vi "Refresh with loaded ROI_retd.vi"(7 "ROI fit info cluster":T1 {"ROI fit info"."Frame size"."Old" items=["100X100"=100, "128X128"=128, "200X200"=200, "256X256"=256, "512X512"=512, "1024x1024"=1024, "2048x2048"=2048]; "ROI fit info"."Frame size"."New" items=["100X100"=100, "128X128"=128, "200X200"=200, "256X256"=256, "512X512"=512, "1024x1024"=1024, "2048x2048"=2048]}, 10 "Old ROI file's data":dbl[][](array[numeric]), 11 "Old ROI file path":path) -> (1 "Last ROI Enum":T3, 3 "Proceed?":bool)   [LabVIEW 2017]
uses:
  Typedefs/ROI ID Enum.ctl
  Typedefs/ROI management FG states.ctl
  Typedefs/Frame Size.ctl
  Typedefs/ROI fitting info cluster.ctl
panel:
  out "No ROI":bool
  out "Number of ROI":i32
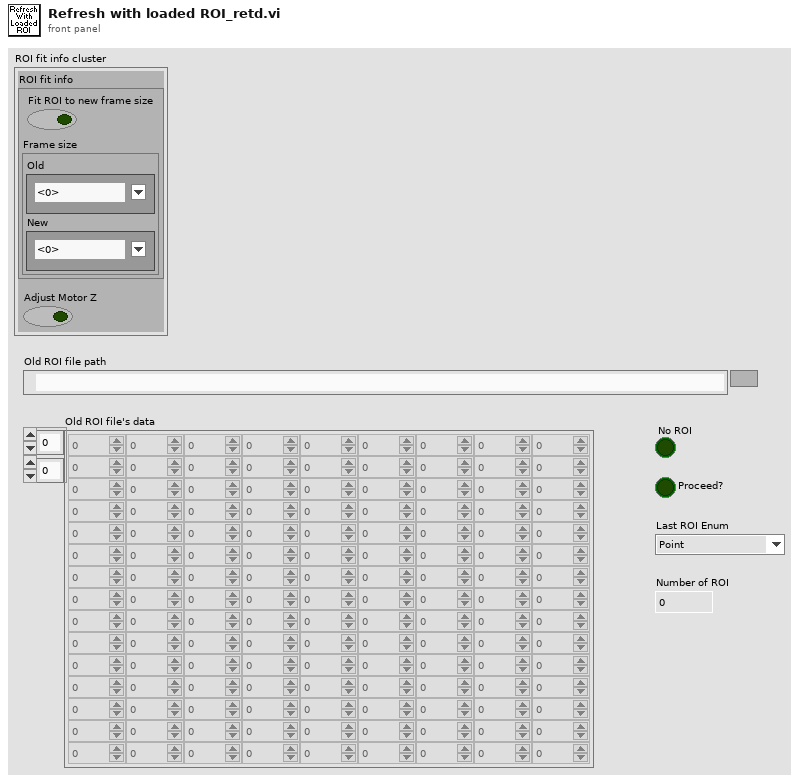
[diagram p1: front panel]
types:
  T1 = typedef "ROI fitting info cluster.ctl" = cluster{"ROI fit info":cluster{"Fit ROI to new frame size":bool, "Frame size":cluster{"Old":T2, "New":T2}}, "Adjust Motor Z":bool}
  T2 = typedef "Frame Size.ctl" = u16
  T3 = typedef "ROI ID Enum.ctl" = enum16{"Point", "MiniScan", "Comp. MiniScan", "Rectangle", "Comp. volume", "Arb. plane point"}
  T4 = typedef "ROI management FG states.ctl" = enum16{"Read", "Write", "Clear Last", "Clear All", "Update ROIs time", "Reload last ROI set", "Offset all ROI", "Offset visible ROI"}
  T5 = typedef "ROI spec.ctl" = cluster{"Coordinates":i32[], "Zoom":dbl, "ROI Enum":T3, "ZplaneIndex":i32}
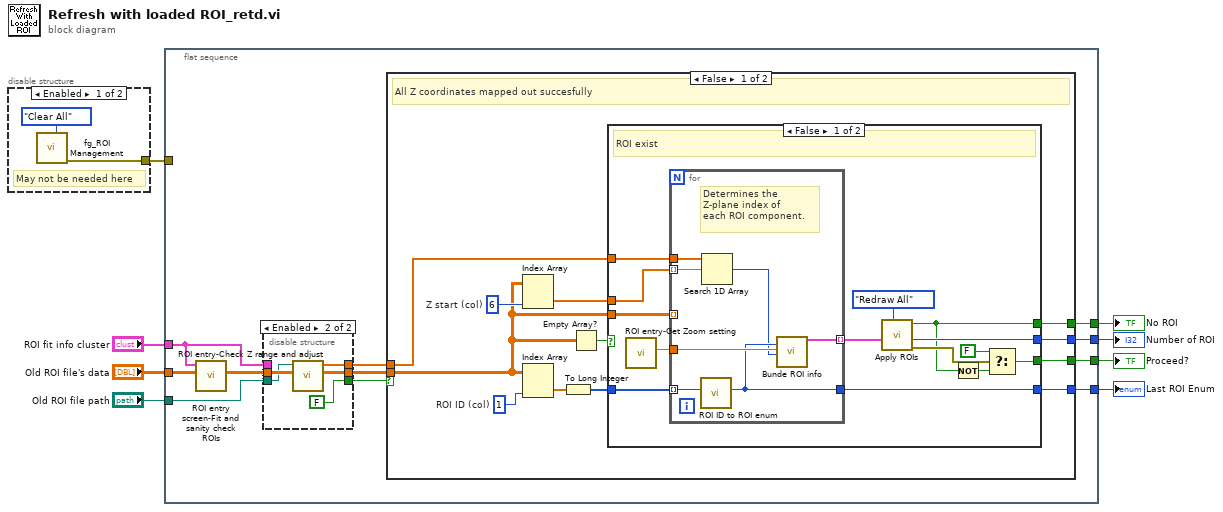
[diagram p0: block diagram]
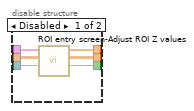
[diagram p2: hidden frame]
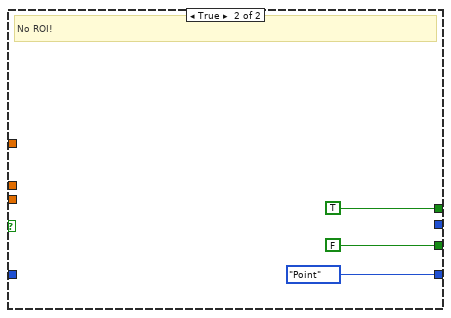
[diagram p3: hidden frame]
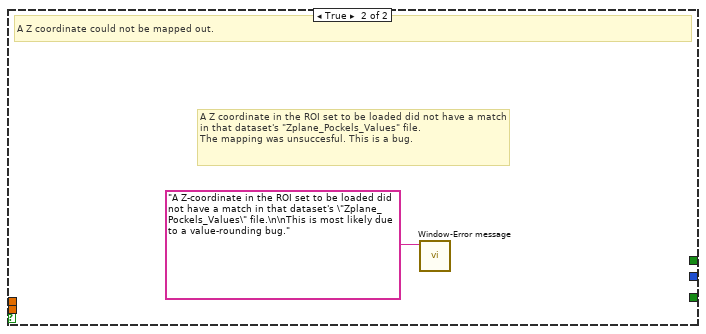
[diagram p4: hidden frame]
diagram:
  n1 = disable-structure shown="Enabled" {
    disable-tunnel: [w9 _] -> w1
    frame Enabled {
      # "May not be needed here"
      n2 = call "fg_ROI Management.vi"("Function"=ROI_management_FG_states."Clear All") -> ("error out"=w9:errorcluster)  [unwired: 6 in, 4 out]
    }
    frame Disabled {
    }
  }
  n3 = flat-sequence {
    tunnel: "Old ROI file path" -> [w13]
    tunnel: [w21] -> w7
    tunnel: [w20] -> w6
    tunnel: [w19] -> w5
    tunnel: [w18] -> w4
    tunnel: "Old ROI file's data" -> [w17]
    tunnel: "ROI fit info cluster" -> [w14]
    tunnel: w1 -> [_]
    frame #0 {
      n4 = call "ROI entry screen-Fit and sanity check ROIs.vi"("Old ROI file's data in"=w17, "ROI fit info"=w14) -> ("Fitted ROI data"=w16:dbl[][])  [unwired: 9 in]
      n5 = disable-structure shown="Enabled" {
        disable-tunnel: w16 -> [w27 w32]
        disable-tunnel: [w26 w29] -> w15
        disable-tunnel: w14 -> [w25 _]
        disable-tunnel: w13 -> [w24 w31]
        disable-tunnel: [w23 w30] -> w12
        disable-tunnel: [w22 FALSE ("A Z coordinate could not be mapped")] -> w11
        frame Disabled {
          n6 = call "ROI entry screen-Adjust ROI Z values.vi"("Old ROI file path"=w24, "Old ROI file's data in"=w27, "ROI fit info"=w25) -> ("A Z coordinate could not be mapped"=w22:bool, "Fitted ROI data"=w26:dbl[][], "Latest AOL Z (um)"=w23:dbl[])  [unwired: 6 in]
        }
        frame Enabled {
          n7 = call "ROI entry-Check Z range and adjust.vi"("ROI File data"=w32, "Old ROI file path"=w31) -> ("Adjusted ROI Data"=w29:dbl[][], "Latest AOL Z values"=w30:dbl[])  [unwired: 8 in]
        }
      }
      n8 = case shown="False" w11 {
        tunnel: [w44 _] -> w21
        tunnel: [w43 _] -> w20
        tunnel: [w42 _] -> w19
        tunnel: [w41 _] -> w18
        tunnel: w15 -> [w34 _]
        tunnel: w12 -> [w33 _]
        frame False {
          w37 = 1  # ROI ID (col)
          w38 = 6  # Z start (col)
          # "All Z coordinates mapped out succesfully"
          n9 = Index Array(array=w34, index (col)=w38) -> (element=w39:dbl[])  [unwired: 1 in]
          n10 = Index Array(array=w34, index (col)=w37) -> (element=w36:dbl[])  [unwired: 1 in]
          n11 = To Long Integer(number=w36) -> (32bit integer=w40:i32[])
          n12 = Empty Array?(array=w34) -> (empty?=w35:bool)
          n13 = case shown="False" w35 {
            tunnel: w34 -> [w47 _]
            tunnel: [w49 ROI_ID_Enum."Point" ("ROI Enum")] -> w43
            tunnel: [w55 FALSE ("Proceed?")] -> w44
            tunnel: [w53 _] -> w42
            tunnel: [w52 TRUE ("No ROI")] -> w41
            tunnel: w40 -> [w50 _]
            tunnel: w39 -> [w46 _]
            tunnel: w33 -> [w45 _]
            frame False {
              # "ROI exist"
              n14 = call "ROI entry-Get Zoom setting.vi"() -> ("Zoom Value"=w54:dbl)  [unwired: 9 in, 2 out]
              n15 = for {
                tunnel: w47 -> [_] mode=indexing
                tunnel: [w66] -> w58 mode=indexing
                tunnel: w54 -> [w64]
                tunnel: w50 -> [w63] mode=indexing
                tunnel: [w62] -> w49
                tunnel: w46 -> [w60] mode=indexing
                tunnel: w45 -> [w61]
                # "Determines the\nZ-plane index of\neach ROI component."
                n16 = call "ROI ID to ROI enum.vi"("ROI ID"=w63) -> ("ROI Enum"=w62:T3)  [unwired: 6 in]
                n17 = Search 1D Array(1D array=w61, element=w60) -> (index of element=w59:i32)  [unwired: 1 in]
                n18 = call "Bunde ROI info.vi"("ROI Enum"=w62, "Zoom"=w64, "ZplaneIndex"=w59) -> ("ROI Coordinates"=w65:i32[], "ROI Info"=w66:T5)  [unwired: 15 in]
              }
              n19 = call "Apply ROIs.vi"("Mode (Redraw All)"=enum16{"Redraw All", "Draw Last"}."Redraw All", "ROIs Info []"=w58) -> ("error out"=w56:errorcluster, "Number of ROI"=w53:i32, "No ROI"=w52:bool)  [unwired: 6 in, 1 out]
              n20 = Not(x=w52) -> (.not. x?=w51:bool)
              n21 = Select(t=FALSE, s=w56, f=w51) -> (s? t:f=w55:bool)
            }
            frame True {
              # "No ROI!"
            }
          }
        }
        frame True {
          # "A Z coordinate in the ROI set to be loaded did not have a match in that dataset's \"Zplane_Pockels_Values\" file.\nThe mapping was unsuccesful. This is a bug."
          # "A Z coordinate could not be mapped out."
          n22 = call "Window-Error message.vi"("Message"="A Z-coordinate in the ROI set to be loaded did not have a match in that dataset's \"Zplane_Pockels_Values\" file.\n\nThis is most likely due to a value-rounding bug.") -> ()  [unwired: 10 in, 1 out]
        }
      }
    }
  }
  "Proceed?" <- w7
  "Last ROI Enum" <- w6
  "Number of ROI" <- w5
  "No ROI" <- w4
